vi "Grid_draw_test.vi"() -> ()   [LabVIEW 2020]
uses:
  <vilib>/GPower/Array/Library/Create/Random/CreateRandomI8.vi
  <vilib>/GPower/Numeric/Library/Random.vi
  <vilib>/GPower/Numeric/Library/Rand/RandI8.vi
  <vilib>/GPower/Array/GPArray.lvlib
panel:
  out "Image Out":T1(plugin-control)
  in  "Grid Lines":i32=2
  in  "N":i32=512
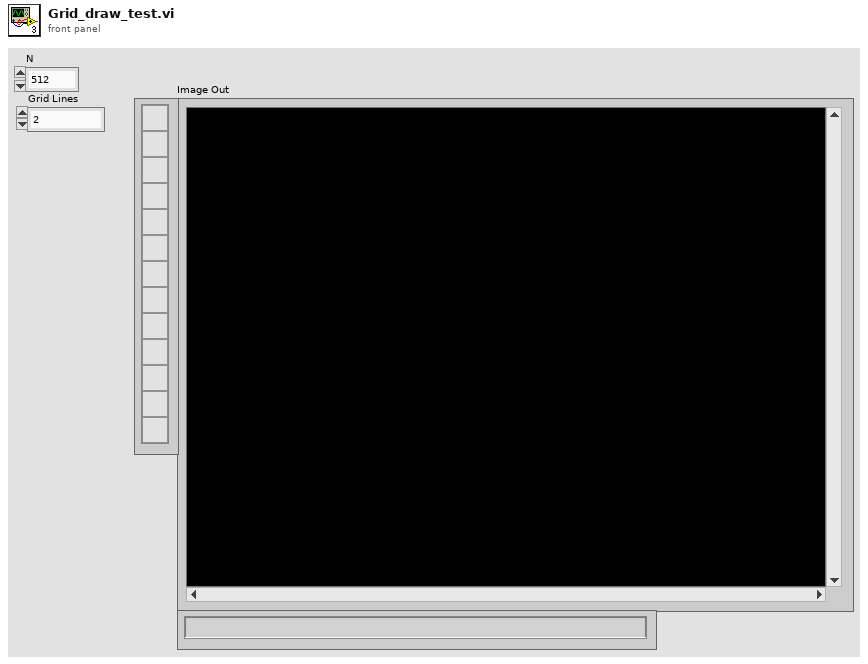
[diagram p1: front panel]
types:
  T1 = typedef "IMAQ Image.ctl" = refnum<image>
  T2 = typedef "Image Type" = u32
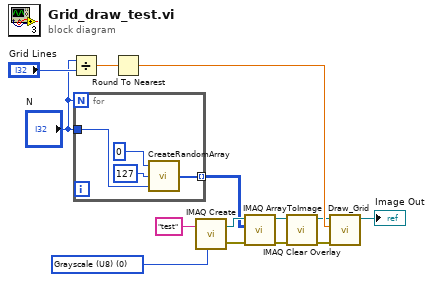
[diagram p0: block diagram]
diagram:
  w13 = T2 0 items=["Grayscale (U8)", "Grayscale (I16)", "Grayscale (SGL)", "Complex (CSG)", "RGB (U32)", "HSL (U32)", "RGB (U64)", "Grayscale (U16)"] ("Image Type")
  n1 = Divide(x="N", y="Grid Lines") -> (x/y=w7:dbl)
  n2 = for {
    N: "N" -> [_]
    tunnel: [w16] -> w10 mode=indexing
    tunnel: "N" -> [w15]
    n3 = call-poly <vilib>:"CreateRandomArray.vi"("N"=w15, "Maximum value"=i8 127, "Minimum value"=i8 0) -> ("Created array"=w16:i8[])
  }
  n4 = Round To Nearest(number=w7) -> (nearest integer value=w6:dbl)
  n5 = call "IMAQ Create"("Image Name"="test", "Image Type"=w13) -> ("New Image"=w11:T1, "error out"=w12:errorcluster)  [unwired: 3 in]
  n6 = call "IMAQ ArrayToImage"("error in (no error)"=w12, "Image Pixels (U8)"=w10, "Image"=w11) -> ("error out"=w1:errorcluster, "Image Out"=w4:T1)  [unwired: 7 in]
  n7 = call "IMAQ Clear Overlay"("error in (no error)"=w1, "Image"=w4) -> ("error out"=w2:errorcluster, "Image Out"=w3:T1)  [unwired: 8 in]
  n8 = call "Draw_Grid.vi"("error in (no error)"=w2, "Grid Lines"=w6, "Image In"=w3) -> ("Image Out"=→"Image Out":T1)  [unwired: 7 in, 1 out]
